vi "currentnumber.vi"() -> ()   [LabVIEW 2011]
panel:
  out "current number":i32
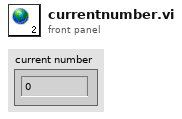
[diagram p1: front panel]
diagram:
